vi "Pop Button back up.vi"(8 "error in (no error)":errorcluster, 11 "Boolean in":refnum<vi>) -> (0 "error out":errorcluster)   [LabVIEW 2024]
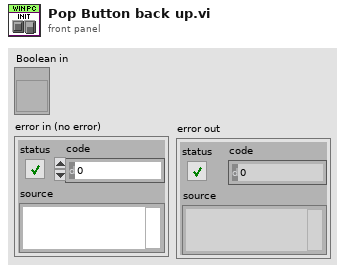
[diagram p1: front panel]
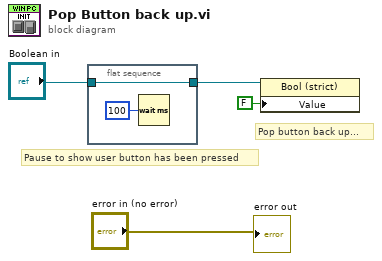
[diagram p0: block diagram]
diagram:
  # "Pause to show user button has been pressed"
  # "Pop button back up..."
  n1 = flat-sequence {
    tunnel: [w5] -> w4
    tunnel: "Boolean in" -> [w5]
    frame #0 {
      n2 = Wait (ms)(milliseconds to wait=u32 100) -> ()  [unwired: 1 out]
    }
  }
  n3 = property class="Bool (strict)"(reference=w4, "Value"=FALSE) -> ()  [unwired: 1 in, 2 out]
  "error out" <- "error in (no error)"
